vi "Main Page.vi"(8 "error in (no error)":errorcluster, 11 "Node Ptr":T1 format="%.0x") -> (0 "error out":errorcluster)   [LabVIEW 2014, in "CAN Bus Monitor System Explorer.lvlib"]
uses:
  CAN Bus Monitor System Explorer.lvlib
  <vilib>/NI Veristand/Custom Device API/Custom Device Item Ref.ctl
  Shared/Constants.vi
  <vilib>/NI Veristand/Custom Device API/Get Item Property (String).vi
  <vilib>/NI Veristand/Custom Device API/Get Item Property (U32).vi
  <vilib>/NI Veristand/Custom Device API/Set Item Property (String).vi
  <vilib>/NI Veristand/Custom Device API/Set Item Property (U32).vi
  <vilib>/NI Veristand/Custom Device API/Custom Device API.lvlib
  Shared/CAN Bus Monitor Shared.lvlib
panel:
  in  "Baud Rate [Bd]":u32
  in  "CAN Port Name (ex: CAN1)":string
  in  "Header":cluster{"Section Name":string}={"Section Name"="Custom Device Item Settings"}
  in  "Description":string
  in  "Name":string
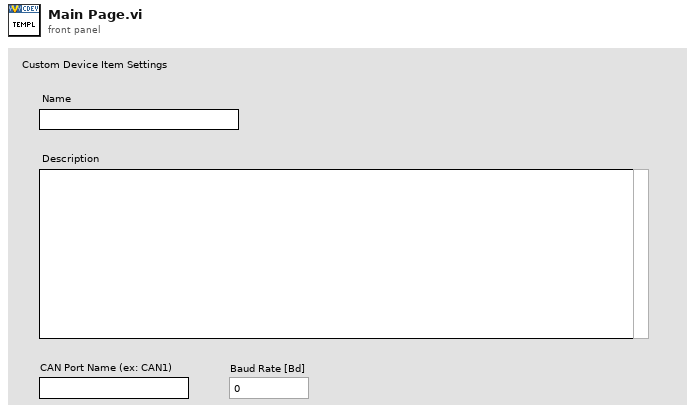
[diagram p1: front panel]
types:
  T1 = typedef "Custom Device API.lvlib/Custom Device Item Ref.ctl" = u64
  T2 = typedef "Custom Device API.lvlib/Custom Device Item Info.ctl" = cluster{"Name":string, "Is Channel":bool, "GUID":string, "Is Waveform":bool}
  T3 = typedef "Custom Device API.lvlib/Custom Device Commands.ctl" = enum16{"Default", "Item renamed", "Shutdown", "Dynamic button pressed"}
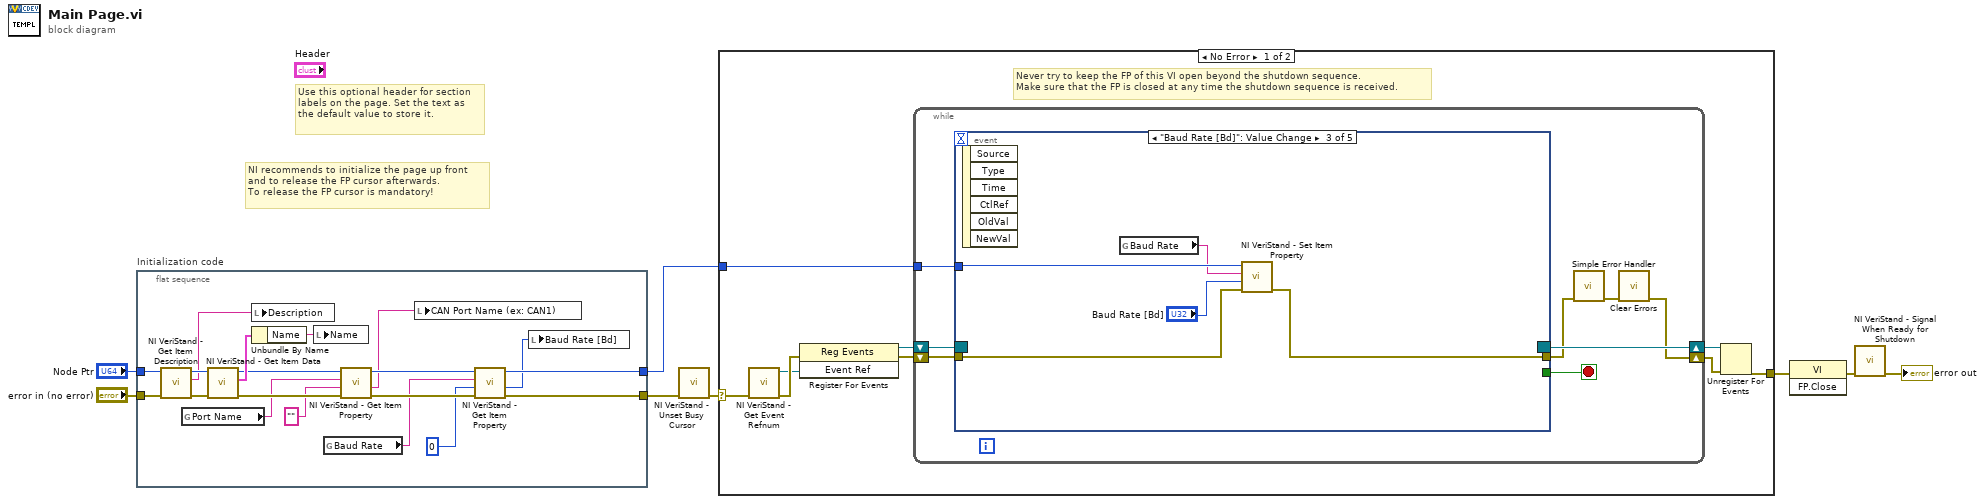
[diagram p0: block diagram]
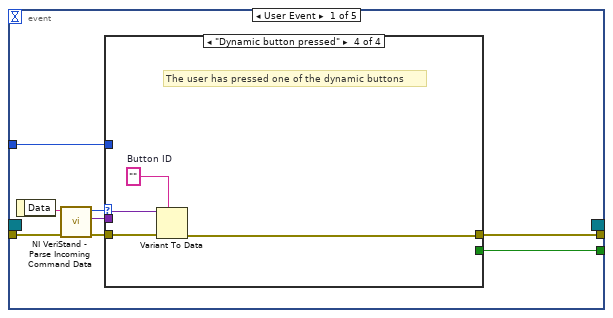
[diagram p2: hidden frame]
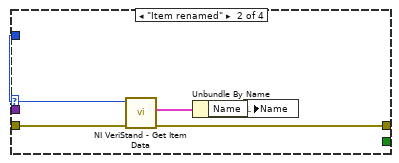
[diagram p4: hidden frame]
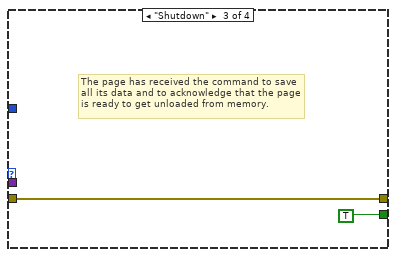
[diagram p5: hidden frame]
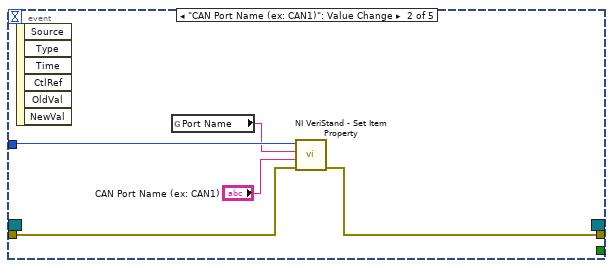
[diagram p6: hidden frame]
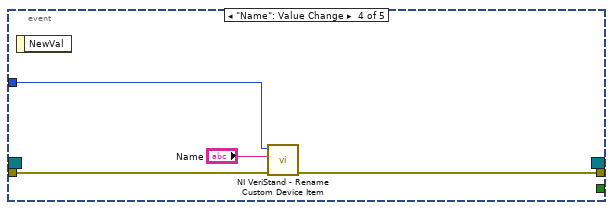
[diagram p7: hidden frame]
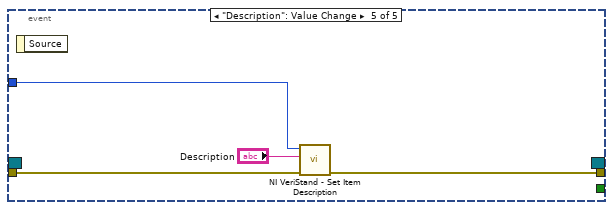
[diagram p8: hidden frame]
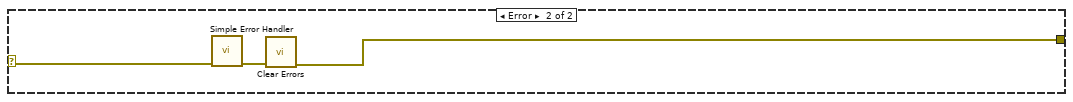
[diagram p9: hidden frame]
diagram:
  # "Use this optional header for section labels on the page. Set the text as the default value to store it."
  # "NI recommends to initialize the page up front\nand to release the FP cursor afterwards.\nTo release the FP cursor is mandatory!"
  n1 = flat-sequence "Initialization code" {
    tunnel: "error in (no error)" -> [w26]
    tunnel: "Node Ptr" -> [w25]
    tunnel: [w17] -> w4
    tunnel: [w15] -> w1
    frame #0 {
      n2 = call <vilib>:"NI VeriStand - Get Item Description.vi"("error in (no error)"=w26, "Item Ref in"=w25) -> ("error out"=w24:errorcluster, "Description"=w20:string, "Item Ref out"=w27:T1)  [unwired: 7 out]
      n3 = global read "Constants.vi" "Port Name"() -> (w14:string)
      n4 = call <vilib>:"NI VeriStand - Get Item Data.vi"("error in (no error)"=w24, "Item Ref in"=w27) -> ("error out"=w22:errorcluster, "Item Info"=w23:T2, "Item Ref out"=w18:T1)  [unwired: 7 out]
      n5 = local write "Description"(w20) -> ()
      n6 = Unbundle By Name(w23) -> ("Name"=w21:string)
      n7 = local write "Name"(w21) -> ()
      n8 = global read "Constants.vi" "Baud Rate"() -> (w11:string)
      n9 = call-poly <vilib>:"NI VeriStand - Get Item Property.vi"("error in (no error)"=w22, "Default Value"="", "Property Name"=w14, "Item Ref in"=w18) -> ("error out"=w19:errorcluster, "Value"=w12:string, "Item Ref out"=w16:T1)  [unwired: 4 in, 1 out]
      n10 = local write "CAN Port Name (ex: CAN1)"(w12) -> ()
      n11 = call-poly <vilib>:"NI VeriStand - Get Item Property.vi"("error in (no error)"=w19, "Default Value"=u32 0, "Property Name"=w11, "Item Ref in"=w16) -> ("error out"=w17:errorcluster, "Value"=w9:u32, "Item Ref out"=w15:T1)  [unwired: 4 in, 1 out]
      n12 = local write "Baud Rate [Bd]"(w9) -> ()
    }
  }
  n13 = call <vilib>:"NI VeriStand - Unset Busy Cursor.vi"("error in (no error)"=w4) -> ("error out"=w3:errorcluster)  [unwired: 10 out]
  n14 = case shown="No Error" w3 {
    selector: w3 -> [w28 w85]
    tunnel: [w33 w83] -> w8
    tunnel: w1 -> [w29 _]
    frame No Error {
      # "Never try to keep the FP of this VI open beyond the shutdown sequence.\nMake sure that the FP is closed at any time the shutdown sequence is received."
      n15 = call <vilib>:"NI VeriStand - Get Event Refnum.vi"("error in (no error)"=w28) -> ("error out"=w36:errorcluster, "Event Ref"=w32:refnum<user-event>)  [unwired: 9 out]
      n16 = register-events(error in=w36, w32) -> (reference out=w30:refnum<event-registration>, error out=w31:errorcluster)  [unwired: 1 in]
      n17 = while {
        tunnel: w29 -> [w40]
        shift-right: [w37] -> w34
        shift-left: w31 -> [w43]
        shift-right: [w44] -> w35
        shift-left: w30 -> [w42]
        stop <- w41 stop-if-true
        n18 = event shown="[2] \"Baud Rate [Bd]\": Value Change" {
          selector: w42 -> [_ _ _ _ _]
          dyn-events: [_ _ _ _ _] -> w44
          timeout: _ -> [_ _ _ _ _]
          tunnel: w43 -> [w52 w68 w73 w78 w81]
          tunnel: [w48 _ _ _ _] -> w41
          tunnel: [w47 w65 w71 w77 w80] -> w39
          tunnel: w40 -> [w46 w69 w74 w76 w82]
          event User Event {
            n19 = event-data() -> ("Data"=w51:string)  [unwired: 1 out]
            n20 = call <vilib>:"NI VeriStand - Parse Incoming Command Data.vi"("error in (no error)"=w52, "Incoming data"=w51) -> ("error out"=w50:errorcluster, "Outgoing data"=w45:variant, "Action"=w49:T3)  [unwired: 7 out]
            n21 = case shown="\"Dynamic button pressed\"" w49 {
              tunnel: w50 -> [w53 w58 w59 w64]
              tunnel: [_ _ TRUE _] -> w48
              tunnel: [w53 w55 w59 w61] -> w47
              tunnel: w46 -> [_ w57 _ _]
              tunnel: w45 -> [_ _ _ w63]
              frame "Default", Default {
              }
              frame "Item renamed" {
                n22 = call <vilib>:"NI VeriStand - Get Item Data.vi"("error in (no error)"=w58, "Item Ref in"=w57) -> ("error out"=w55:errorcluster, "Item Info"=w56:T2)  [unwired: 8 out]
                n23 = Unbundle By Name(w56) -> ("Name"=w54:string)
                n24 = local write "Name"(w54) -> ()
              }
              frame "Shutdown" {
                # "The page has received the command to save all its data and to acknowledge that the page is ready to get unloaded from memory."
              }
              frame "Dynamic button pressed" {
                w62 = ""  # Button ID
                # "The user has pressed one of the dynamic buttons"
                n25 = Variant To Data(error in=w64, type=w62, Variant=w63) -> (error out=w61:errorcluster)  [unwired: 1 out]
              }
            }
          }
          event "CAN Port Name (ex: CAN1)": Value Change {
            n26 = event-data() -> ()  [unwired: 7 out]
            n27 = global read "Constants.vi" "Port Name"() -> (w67:string)
            n28 = call-poly <vilib>:"NI VeriStand - Set Item Property.vi"("error in (no error)"=w68, "Value"="CAN Port Name (ex: CAN1)", "Property Name"=w67, "Item Ref in"=w69) -> ("error out"=w65:errorcluster)  [unwired: 5 in, 2 out]
          }
          event "Baud Rate [Bd]": Value Change {
            n29 = event-data() -> ()  [unwired: 7 out]
            n30 = global read "Constants.vi" "Baud Rate"() -> (w72:string)
            n31 = call-poly <vilib>:"NI VeriStand - Set Item Property.vi"("error in (no error)"=w73, "Value"="Baud Rate [Bd]", "Property Name"=w72, "Item Ref in"=w74) -> ("error out"=w71:errorcluster)  [unwired: 5 in, 2 out]
          }
          event "Name": Value Change {
            n32 = event-data() -> ()  [unwired: 2 out]
            n33 = call <vilib>:"NI VeriStand - Rename Custom Device Item.vi"("error in (no error)"=w78, "New Name"="Name", "Item Ref in"=w76) -> ("error out"=w77:errorcluster)  [unwired: 1 in, 7 out]
          }
          event "Description": Value Change {
            n34 = event-data() -> ()  [unwired: 2 out]
            n35 = call <vilib>:"NI VeriStand - Set Item Description.vi"("error in (no error)"=w81, "Description"="Description", "Item Ref in"=w82) -> ("error out"=w80:errorcluster)  [unwired: 8 out]
          }
        }
        n36 = call <vilib>:"Simple Error Handler.vi"("error in (no error)"=w39) -> ("error out"=w38:errorcluster)  [unwired: 1 in, 7 out]
        n37 = call <vilib>:"Clear Errors.vi"("error in (no error)"=w38) -> ("error out"=w37:errorcluster)  [unwired: 1 in, 5 out]
      }
      n38 = Unregister For Events(event registration refnum=w35, error in=w34) -> (error out=w33:errorcluster)
    }
    frame Error {
      n39 = call <vilib>:"Simple Error Handler.vi"("error in (no error)"=w85) -> ("error out"=w84:errorcluster)  [unwired: 1 in, 7 out]
      n40 = call <vilib>:"Clear Errors.vi"("error in (no error)"=w84) -> ("error out"=w83:errorcluster)  [unwired: 1 in, 5 out]
    }
  }
  n41 = invoke class="VI" method="FP.Close"(error in=w8) -> (error out=w7:errorcluster)  [unwired: 2 in, 2 out]
  n42 = call <vilib>:"NI VeriStand - Signal When Ready for Shutdown.vi"("error in (no error)"=w7) -> ("error out"=→"error out":errorcluster)  [unwired: 10 out]
